vi "Calcolo Errori Medio e Max.vi"(0 "Misure Errore Ampiezza[%]":dbl[](array[numeric]), 1 "Misure Errore Frequenza[mHz]":dbl[](array[numeric]), 4 "Misure Errore Fase[crad]":dbl[](array[numeric]), 5 "Misure Errore TVE[%]":dbl[](array[numeric])) -> (12 "Errore Medio TVE[%]":dbl, 13 "Errore max TVE[%]":dbl, 14 "Errore Medio Ampiezza[%]":dbl, 15 "Errore max Ampiezza[%]":dbl, 16 "Errore Medio Frequenza [mHz]":dbl, 17 "Errore max Frequenza [mHz]":dbl, 18 "Errore Medio Fase[crad]":dbl, 19 "Errore max Fase[crad]":dbl)   [LabVIEW 2019]
uses:
  <vilib>/Analysis/baseanly.llb/Mean (DBL).vi
  <vilib>/Analysis/NI_AALBase.lvlib
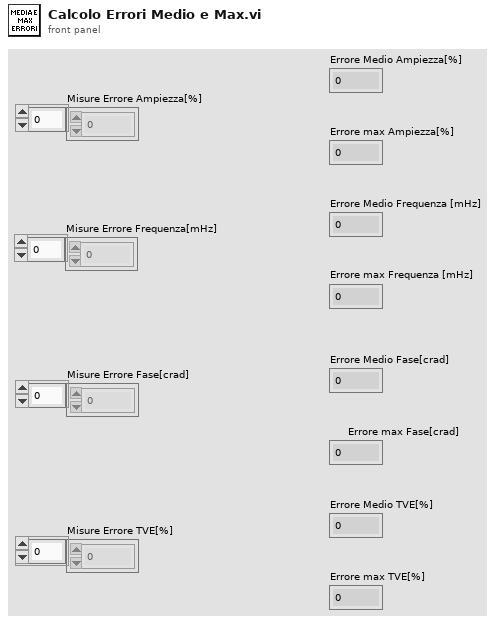
[diagram p1: front panel]
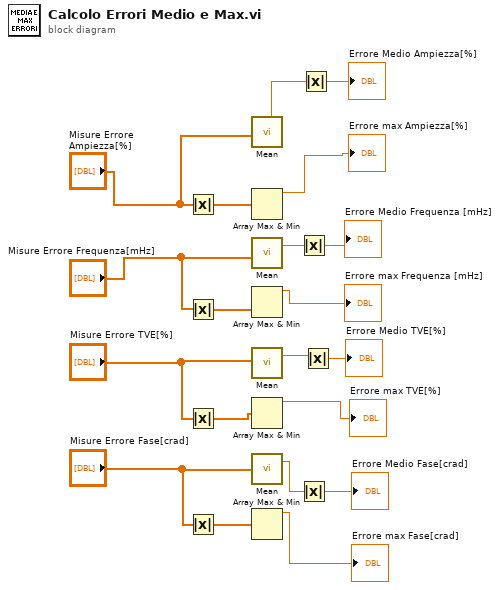
[diagram p0: block diagram]
diagram:
  n1 = Absolute Value(x="Misure Errore Ampiezza[%]") -> (abs(x)=w10:dbl[])
  n2 = Absolute Value(x="Misure Errore Frequenza[mHz]") -> (abs(x)=w12:dbl[])
  n3 = Absolute Value(x="Misure Errore TVE[%]") -> (abs(x)=w14:dbl[])
  n4 = Absolute Value(x="Misure Errore Fase[crad]") -> (abs(x)=w16:dbl[])
  n5 = call-poly <vilib>:"Mean.vi"("X"="Misure Errore Ampiezza[%]") -> ("mean"=w2:dbl)  [unwired: 1 out]
  n6 = Array Max & Min(array=w10) -> (max value=→"Errore max Ampiezza[%]":dbl)  [unwired: 3 out]
  n7 = call-poly <vilib>:"Mean.vi"("X"="Misure Errore Frequenza[mHz]") -> ("mean"=w4:dbl)  [unwired: 1 out]
  n8 = Array Max & Min(array=w12) -> (max value=→"Errore max Frequenza [mHz]":dbl)  [unwired: 3 out]
  n9 = call-poly <vilib>:"Mean.vi"("X"="Misure Errore TVE[%]") -> ("mean"=w6:dbl)  [unwired: 1 out]
  n10 = Array Max & Min(array=w14) -> (max value=→"Errore max TVE[%]":dbl)  [unwired: 3 out]
  n11 = call-poly <vilib>:"Mean.vi"("X"="Misure Errore Fase[crad]") -> ("mean"=w8:dbl)  [unwired: 1 out]
  n12 = Array Max & Min(array=w16) -> (max value=→"Errore max Fase[crad]":dbl)  [unwired: 3 out]
  n13 = Absolute Value(x=w4) -> (abs(x)=→"Errore Medio Frequenza [mHz]":dbl)
  n14 = Absolute Value(x=w8) -> (abs(x)=→"Errore Medio Fase[crad]":dbl)
  n15 = Absolute Value(x=w2) -> (abs(x)=→"Errore Medio Ampiezza[%]":dbl)
  n16 = Absolute Value(x=w6) -> (abs(x)=→"Errore Medio TVE[%]":dbl)
